vi "digWaveFromPlatData.vi"() -> ()   [LabVIEW 2017]
uses:
  <vilib>/Waveform/DWDTOps.llb/DWDT Digital to Binary U8.vi
  <vilib>/DAQmx/write.llb/DAQmx Write (Digital 2D U8 NChan NSamp).vi
  <vilib>/DAQmx/configure/timing.llb/DAQmx Timing (Sample Clock).vi
  <vilib>/DAQmx/create/channels.llb/DAQmx Create Channel (DO-Digital Output).vi
  <vilib>/Waveform/DWDTOps.llb/DWDT Boolean Array to Digital.vi
panel:
  out "Digital Waveform Graph 2":digitalwaveform(graph)
  out "Digital Waveform Graph":digitalwaveform(graph)
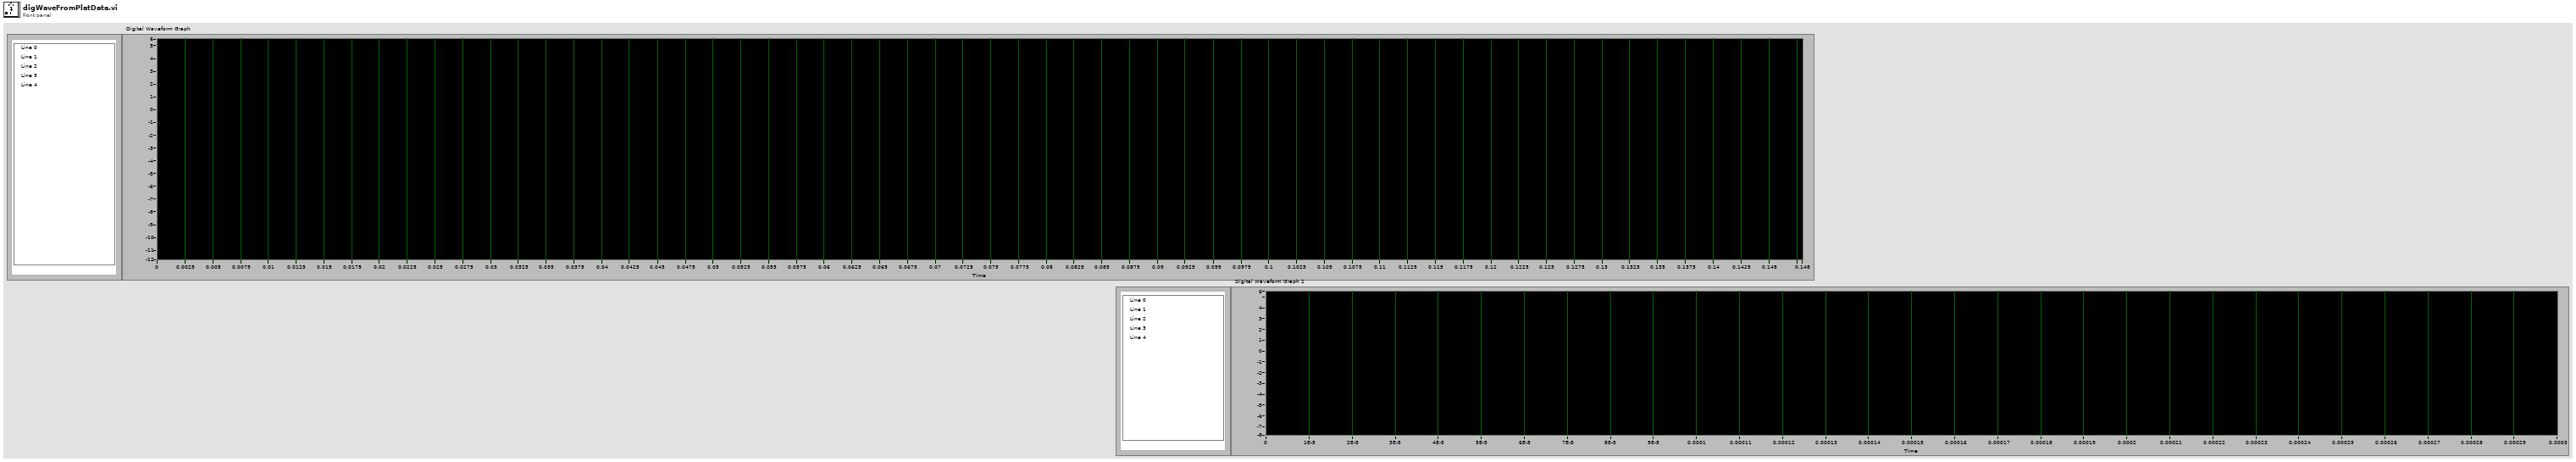
[diagram p1: front panel]
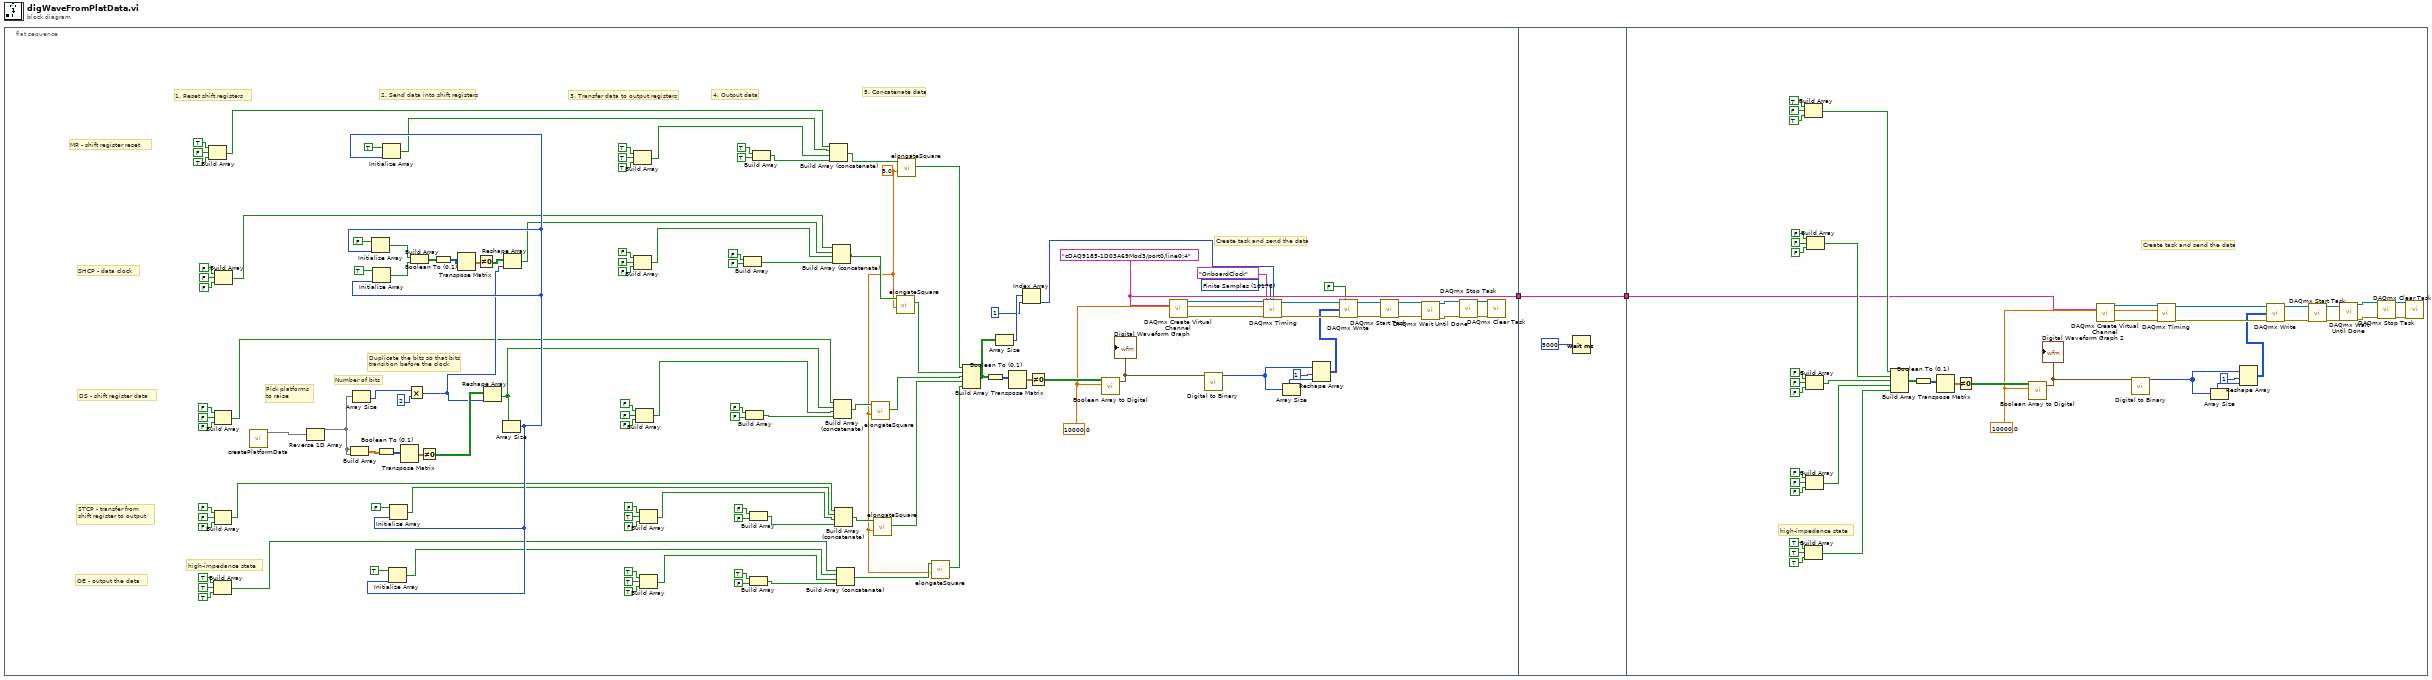
[diagram p0: block diagram]
diagram:
  n1 = flat-sequence {
    tunnel: [w26] -> w1
    tunnel: [w125] -> w2
    tunnel: w1 -> [w125]
    tunnel: w2 -> [w132]
    frame #0 {
      w4 = 5.0 ("concatenation \nfactor")
      w25 = 10178 items=["Finite Samples"=10178, "Continuous Samples"=10123, "Hardware Timed Single Point"=12522] ("sample mode")
      w26 = tag "cDAQ9185-1D03A69Mod3/port0/line0:4" ("lines")
      w36 = 10000.0 ("rate")
      # "Create task and send the data"
      # "5. Concatenate data"
      # "4. Output data"
      # "3. Transfer data to output registers"
      # "2. Send data into shift registers"
      # "Duplicate the bits so that bits \ntransition before the clock"
      # "Pick platforms \nto raise"
      # "Number of bits"
      # "high-impedance state"
      # "OE - output the data"
      # "STCP - transfer from \nshift register to output"
      # "DS - shift register data"
      # "MR - shift register reset"
      # "SHCP - data clock"
      # "1. Reset shift registers"
      n2 = Build Array(TRUE, FALSE, TRUE) -> (w63:bool[])
      n3 = Build Array(TRUE, TRUE, TRUE) -> (w47:bool[])
      n4 = Build Array(FALSE, FALSE, FALSE) -> (w55:bool[])
      n5 = Build Array(FALSE, FALSE, FALSE) -> (w51:bool[])
      n6 = Build Array(FALSE, FALSE, FALSE) -> (w59:bool[])
      n7 = call "createPlatformData.vi"() -> (3:w3)  [unwired: 11 in]
      n8 = Reverse 1D Array(array=w3) -> (reversed array=w74:ext[])
      n9 = Build Array(w74, w74) -> (w106:ext[][])
      n10 = Array Size(array=w74) -> (size(s)=w108:i32)
      n11 = Boolean To (0,1)(Boolean=w106) -> (0, 1=w105:i16[][])
      n12 = Transpose Matrix(1:w105) -> (0:w104:dbl[][])
      n13 = Multiply(x=w108, y=2) -> (x*y=w81:i32)
      n14 = Not Equal To 0?(x=w104) -> (x != 0?=w103:bool[][])
      n15 = Reshape Array(w103, w81) -> (w54:bool[])
      n16 = Array Size(array=w54) -> (size(s)=w88:i32)
      n17 = Initialize Array(FALSE, w88) -> (w87:bool[])
      n18 = Initialize Array(TRUE, w88) -> (w86:bool[])
      n19 = Initialize Array(TRUE, w88) -> (w62:bool[])
      n20 = Initialize Array(TRUE, w88) -> (w46:bool[])
      n21 = Initialize Array(FALSE, w88) -> (w50:bool[])
      n22 = Build Array(w87, w86) -> (w85:bool[][])
      n23 = Boolean To (0,1)(Boolean=w85) -> (0, 1=w84:i16[][])
      n24 = Transpose Matrix(1:w84) -> (0:w83:dbl[][])
      n25 = Not Equal To 0?(x=w83) -> (x != 0?=w82:bool[][])
      n26 = Reshape Array(w82, w81) -> (w58:bool[])
      n27 = Build Array(TRUE, TRUE, TRUE) -> (w61:bool[])
      n28 = Build Array(FALSE, FALSE, FALSE) -> (w57:bool[])
      n29 = Build Array(FALSE, FALSE, FALSE) -> (w53:bool[])
      n30 = Build Array(FALSE, TRUE, FALSE) -> (w49:bool[])
      n31 = Build Array(TRUE, TRUE, TRUE) -> (w45:bool[])
      n32 = Build Array(FALSE, FALSE) -> (w56:bool[])
      n33 = Build Array(FALSE, FALSE) -> (w52:bool[])
      n34 = Build Array(FALSE, FALSE) -> (w48:bool[])
      n35 = Build Array(TRUE, FALSE) -> (w44:bool[])
      n36 = Build Array(TRUE, TRUE) -> (w60:bool[])
      n37 = Build Array (concatenate)(w63, w62, w61, w60) -> (w14:bool[])
      n38 = Build Array (concatenate)(w59, w58, w57, w56) -> (w12:bool[])
      n39 = Build Array (concatenate)(w55, w54, w53, w52) -> (w10:bool[])
      n40 = Build Array (concatenate)(w51, w50, w49, w48) -> (w8:bool[])
      n41 = Build Array (concatenate)(w47, w46, w45, w44) -> (w6:bool[])
      n42 = call "elongateSquare.vi"("concatenation \nfactor"=w4, "Array"=w10) -> ("catVector"=w9:bool[])  [unwired: 9 in]
      n43 = call "elongateSquare.vi"("concatenation \nfactor"=w4, "Array"=w8) -> ("catVector"=w7:bool[])  [unwired: 9 in]
      n44 = call "elongateSquare.vi"("concatenation \nfactor"=w4, "Array"=w12) -> ("catVector"=w11:bool[])  [unwired: 9 in]
      n45 = call "elongateSquare.vi"("concatenation \nfactor"=w4, "Array"=w14) -> ("catVector"=w13:bool[])  [unwired: 9 in]
      n46 = call "elongateSquare.vi"("concatenation \nfactor"=w4, "Array"=w6) -> ("catVector"=w5:bool[])  [unwired: 9 in]
      n47 = Build Array(w13, w11, w9, w7, w5) -> (w23:bool[][])
      n48 = Boolean To (0,1)(Boolean=w23) -> (0, 1=w43:i16[][])
      n49 = Array Size(array=w23) -> (size(s)=w22:i32[])
      n50 = Transpose Matrix(1:w43) -> (0:w42:dbl[][])
      n51 = Index Array(array=w22, index=1) -> (element=w19:i32)
      n52 = Not Equal To 0?(x=w42) -> (x != 0?=w41:bool[][])
      n53 = call-poly <vilib>:"Boolean Array to Digital.vi"("sample rate"=w36, "boolean array"=w41) -> ("digital waveform"=w35:digitalwaveform)  [unwired: 8 in, 1 out]
      "Digital Waveform Graph" <- w35
      n54 = call-poly <vilib>:"DAQmx Create Virtual Channel.vi"("lines"=w26) -> ("task out"=w40:refnum<k21>, "error out"=w39:errorcluster)  [unwired: 13 in]
      n55 = call-poly <vilib>:"Digital to Binary.vi"("digital waveform"=w35) -> ("binary array"=w32:u8[])  [unwired: 9 in, 1 out]
      n56 = call-poly <vilib>:"DAQmx Timing.vi"("task/channels in"=w40, "sample mode"=w25, "samples per channel"=w19, "rate"=w36, "source"=tag "OnboardClock", "error in"=w39) -> ("task out"=w38:refnum<k21>, "error out"=w37:errorcluster)  [unwired: 8 in]
      n57 = Array Size(array=w32) -> (size(s)=w31:i32)
      n58 = Reshape Array(w32, 1, w31) -> (w33:u8[][])
      n59 = call-poly <vilib>:"DAQmx Write.vi"("task/channels in"=w38, "auto start"=FALSE, "data"=w33, "error in"=w37) -> ("task out"=w30:refnum<k21>, "error out"=w29:errorcluster)  [unwired: 9 in, 1 out]
      n60 = call <vilib>:"DAQmx Start Task.vi"("task/channels in"=w30, "error in"=w29) -> ("task out"=w18:refnum<k21>, "error out"=w17:errorcluster)  [unwired: 12 in]
      n61 = call <vilib>:"DAQmx Wait Until Done.vi"("task/channels in"=w18, "error in"=w17) -> ("task out"=w16:refnum<k21>, "error out"=w15:errorcluster)  [unwired: 12 in]
      n62 = call <vilib>:"DAQmx Stop Task.vi"("task/channels in"=w16, "error in"=w15) -> ("task out"=w28:refnum<k21>, "error out"=w27:errorcluster)  [unwired: 12 in]
      n63 = call <vilib>:"DAQmx Clear Task.vi"("task in"=w28, "error in"=w27) -> ()  [unwired: 13 in, 1 out]
    }
    frame #1 {
      n64 = Wait (ms)(milliseconds to wait=5000) -> ()  [unwired: 1 out]
    }
    frame #2 {
      w145 = 10000.0 ("rate")
      # "Create task and send the data"
      # "high-impedance state"
      n65 = Build Array(TRUE, FALSE, TRUE) -> (w137:bool[])
      n66 = Build Array(TRUE, TRUE, TRUE) -> (w133:bool[])
      n67 = Build Array(FALSE, FALSE, FALSE) -> (w135:bool[])
      n68 = Build Array(FALSE, FALSE, FALSE) -> (w134:bool[])
      n69 = Build Array(FALSE, FALSE, FALSE) -> (w136:bool[])
      n70 = Build Array(w137, w136, w135, w134, w133) -> (w151:bool[][])
      n71 = Boolean To (0,1)(Boolean=w151) -> (0, 1=w153:i16[][])
      n72 = Transpose Matrix(1:w153) -> (0:w152:dbl[][])
      n73 = Not Equal To 0?(x=w152) -> (x != 0?=w150:bool[][])
      n74 = call-poly <vilib>:"Boolean Array to Digital.vi"("sample rate"=w145, "boolean array"=w150) -> ("digital waveform"=w144:digitalwaveform)  [unwired: 8 in, 1 out]
      "Digital Waveform Graph 2" <- w144
      n75 = call-poly <vilib>:"DAQmx Create Virtual Channel.vi"("lines"=w132) -> ("task out"=w149:refnum<k21>, "error out"=w148:errorcluster)  [unwired: 13 in]
      n76 = call-poly <vilib>:"Digital to Binary.vi"("digital waveform"=w144) -> ("binary array"=w141:u8[])  [unwired: 9 in, 1 out]
      n77 = call-poly <vilib>:"DAQmx Timing.vi"("task/channels in"=w149, "rate"=w145, "error in"=w148) -> ("task out"=w147:refnum<k21>, "error out"=w146:errorcluster)  [unwired: 11 in]
      n78 = Array Size(array=w141) -> (size(s)=w140:i32)
      n79 = Reshape Array(w141, 1, w140) -> (w142:u8[][])
      n80 = call-poly <vilib>:"DAQmx Write.vi"("task/channels in"=w147, "data"=w142, "error in"=w146) -> ("task out"=w139:refnum<k21>, "error out"=w138:errorcluster)  [unwired: 10 in, 1 out]
      n81 = call <vilib>:"DAQmx Start Task.vi"("task/channels in"=w139, "error in"=w138) -> ("task out"=w127:refnum<k21>, "error out"=w126:errorcluster)  [unwired: 12 in]
      n82 = call <vilib>:"DAQmx Wait Until Done.vi"("task/channels in"=w127, "error in"=w126) -> ("task out"=w130:refnum<k21>, "error out"=w131:errorcluster)  [unwired: 12 in]
      n83 = call <vilib>:"DAQmx Stop Task.vi"("task/channels in"=w130, "error in"=w131) -> ("task out"=w128:refnum<k21>, "error out"=w129:errorcluster)  [unwired: 12 in]
      n84 = call <vilib>:"DAQmx Clear Task.vi"("task in"=w128, "error in"=w129) -> ()  [unwired: 13 in, 1 out]
    }
  }
